vi "WILT Start Stop Button Case.vi"(4 "Semaphore":T1[](array[typedef]), 6 "Dryer Step 4 In":T2 {"Night Cycle Count" format="%04d"; "Day Cycle Count" format="%04d"}, 7 "Agilent Valve and Switch Locations":T4[](array[typedef])=[{"Channel"="301", "Station"="1", "Label"="Water Valve", "Agilent Station"="2", "Data"=0.0}, {"Channel"="302", "Station"="2", "Label"="Water Valve", "Agilent Station"="2", "Data"=0.0}, {"Channel"="303", "Station"="3", "Label"="Water Valve", "Agilent Station"="2", "Data"=0.0}, {"Channel"="304", "Station"="4", "Label"="Water Valve", "Agilent Station"="2", "Data"=0.0}, {"Channel"="305", "Station"="5", "Label"="Water Valve", "Agilent Station"="2", "Data"=0.0}, {"Channel"="306", "Station"="6", "Label"="Water Valve", "Agilent Station"="2", "Data"=0.0}, {"Channel"="307", "Station"="7", "Label"="Water Valve", "Agilent Station"="2", "Data"=0.0}, {"Channel"="308", "Station"="8", "Label"="Water Valve", "Agilent Station"="2", "Data"=0.0}, {"Channel"="309", "Station"="9", "Label"="Water Valve", "Agilent Station"="2", "Data"=0.0}, {"Channel"="310", "Station"="10", "Label"="Water Valve", "Agilent Station"="2", "Data"=0.0}, {"Channel"="311", "Station"="11", "Label"="Water Valve", "Agilent Station"="2", "Data"=0.0}, {"Channel"="312", "Station"="12", "Label"="Water Valve", "Agilent Station"="2", "Data"=0.0}, {"Channel"="313", "Station"="13", "Label"="Water Valve", "Agilent Station"="2", "Data"=0.0}, {"Channel"="314", "Station"="14", "Label"="Water Valve", "Agilent Station"="2", "Data"=0.0}, {"Channel"="315", "Station"="15", "Label"="Water Valve", "Agilent Station"="2", "Data"=0.0}, {"Channel"="316", "Station"="16", "Label"="Water Valve", "Agilent Station"="2", "Data"=0.0}, {"Channel"="317", "Station"="17", "Label"="Water Valve", "Agilent Station"="2", "Data"=0.0}, {"Channel"="318", "Station"="18", "Label"="Water Valve", "Agilent Station"="2", "Data"=0.0}, {"Channel"="319", "Station"="19", "Label"="Water Valve", "Agilent Station"="2", "Data"=0.0}, {"Channel"="320", "Station"="20", "Label"="Water Valve", "Agilent Station"="2", "Data"=0.0}, {"Channel"="101", "Station"="21", "Label"="Water Valve", "Agilent Station"="3", "Data"=0.0}, {"Channel"="102", "Station"="22", "Label"="Water Valve", "Agilent Station"="3", "Data"=0.0}, {"Channel"="103", "Station"="23", "Label"="Water Valve", "Agilent Station"="3", "Data"=0.0}, {"Channel"="104", "Station"="24", "Label"="Water Valve", "Agilent Station"="3", "Data"=0.0}, {"Channel"="105", "Station"="25", "Label"="Water Valve", "Agilent Station"="3", "Data"=0.0}, {"Channel"="106", "Station"="26", "Label"="Water Valve", "Agilent Station"="3", "Data"=0.0}, {"Channel"="107", "Station"="27", "Label"="Water Valve", "Agilent Station"="3", "Data"=0.0}, {"Channel"="108", "Station"="28", "Label"="Water Valve", "Agilent Station"="3", "Data"=0.0}, {"Channel"="109", "Station"="29", "Label"="Water Valve", "Agilent Station"="3", "Data"=0.0}, {"Channel"="110", "Station"="30", "Label"="Water Valve", "Agilent Station"="3", "Data"=0.0}, {"Channel"="111", "Station"="31", "Label"="Water Valve", "Agilent Station"="3", "Data"=0.0}, {"Channel"="112", "Station"="32", "Label"="Water Valve", "Agilent Station"="3", "Data"=0.0}, {"Channel"="101", "Station"="33", "Label"="Water Valve", "Agilent Station"="5", "Data"=0.0}, {"Channel"="102", "Station"="34", "Label"="Water Valve", "Agilent Station"="5", "Data"=0.0}, {"Channel"="103", "Station"="35", "Label"="Water Valve", "Agilent Station"="5", "Data"=0.0}, {"Channel"="104", "Station"="36", "Label"="Water Valve", "Agilent Station"="5", "Data"=0.0}, {"Channel"="105", "Station"="37", "Label"="Water Valve", "Agilent Station"="5", "Data"=0.0}, {"Channel"="106", "Station"="38", "Label"="Water Valve", "Agilent Station"="5", "Data"=0.0}, {"Channel"="107", "Station"="39", "Label"="Water Valve", "Agilent Station"="5", "Data"=0.0}, {"Channel"="108", "Station"="40", "Label"="Water Valve", "Agilent Station"="5", "Data"=0.0}, {"Channel"="109", "Station"="41", "Label"="Water Valve", "Agilent Station"="5", "Data"=0.0}, {"Channel"="110", "Station"="42", "Label"="Water Valve", "Agilent Station"="5", "Data"=0.0}, {"Channel"="111", "Station"="43", "Label"="Water Valve", "Agilent Station"="5", "Data"=0.0}, {"Channel"="112", "Station"="44", "Label"="Water Valve", "Agilent Station"="5", "Data"=0.0}, {"Channel"="113", "Station"="45", "Label"="Water Valve", "Agilent Station"="5", "Data"=0.0}, {"Channel"="114", "Station"="46", "Label"="Water Valve", "Agilent Station"="5", "Data"=0.0}, {"Channel"="115", "Station"="47", "Label"="Water Valve", "Agilent Station"="5", "Data"=0.0}, {"Channel"="116", "Station"="48", "Label"="Water Valve", "Agilent Station"="5", "Data"=0.0}, {"Channel"="117", "Station"="49", "Label"="Water Valve", "Agilent Station"="5", "Data"=0.0}, {"Channel"="118", "Station"="50", "Label"="Water Valve", "Agilent Station"="5", "Data"=0.0}, {"Channel"="119", "Station"="51", "Label"="Water Valve", "Agilent Station"="5", "Data"=0.0}, {"Channel"="120", "Station"="52", "Label"="Water Valve", "Agilent Station"="5", "Data"=0.0}, {"Channel"="201", "Station"="53", "Label"="Water Valve", "Agilent Station"="5", "Data"=0.0}, {"Channel"="202", "Station"="54", "Label"="Water Valve", "Agilent Station"="5", "Data"=0.0}, {"Channel"="203", "Station"="55", "Label"="Water Valve", "Agilent Station"="5", "Data"=0.0}, {"Channel"="204", "Station"="56", "Label"="Water Valve", "Agilent Station"="5", "Data"=0.0}, {"Channel"="301", "Station"="21", "Label"="Start Button", "Agilent Station"="5", "Data"=0.0}, {"Channel"="302", "Station"="22", "Label"="Start Button", "Agilent Station"="5", "Data"=0.0}, {"Channel"="303", "Station"="23", "Label"="Start Button", "Agilent Station"="5", "Data"=0.0}, {"Channel"="304", "Station"="24", "Label"="Start Button", "Agilent Station"="5", "Data"=0.0}, {"Channel"="305", "Station"="25", "Label"="Start Button", "Agilent Station"="5", "Data"=0.0}, {"Channel"="306", "Station"="26", "Label"="Start Button", "Agilent Station"="5", "Data"=0.0}, {"Channel"="307", "Station"="27", "Label"="Start Button", "Agilent Station"="5", "Data"=0.0}, {"Channel"="308", "Station"="28", "Label"="Start Button", "Agilent Station"="5", "Data"=0.0}, {"Channel"="309", "Station"="29", "Label"="Start Button", "Agilent Station"="5", "Data"=0.0}, {"Channel"="310", "Station"="30", "Label"="Start Button", "Agilent Station"="5", "Data"=0.0}, {"Channel"="311", "Station"="31", "Label"="Start Button", "Agilent Station"="5", "Data"=0.0}, {"Channel"="312", "Station"="32", "Label"="Start Button", "Agilent Station"="5", "Data"=0.0}, {"Channel"="101", "Station"="33", "Label"="Start Button", "Agilent Station"="7", "Data"=0.0}, {"Channel"="102", "Station"="34", "Label"="Start Button", "Agilent Station"="7", "Data"=0.0}, {"Channel"="103", "Station"="35", "Label"="Start Button", "Agilent Station"="7", "Data"=0.0}, {"Channel"="104", "Station"="36", "Label"="Start Button", "Agilent Station"="7", "Data"=0.0}, {"Channel"="105", "Station"="37", "Label"="Start Button", "Agilent Station"="7", "Data"=0.0}, {"Channel"="106", "Station"="38", "Label"="Start Button", "Agilent Station"="7", "Data"=0.0}, {"Channel"="107", "Station"="39", "Label"="Start Button", "Agilent Station"="7", "Data"=0.0}, {"Channel"="108", "Station"="40", "Label"="Start Button", "Agilent Station"="7", "Data"=0.0}, {"Channel"="109", "Station"="41", "Label"="Start Button", "Agilent Station"="7", "Data"=0.0}, {"Channel"="110", "Station"="42", "Label"="Start Button", "Agilent Station"="7", "Data"=0.0}, {"Channel"="111", "Station"="43", "Label"="Start Button", "Agilent Station"="7", "Data"=0.0}, {"Channel"="112", "Station"="44", "Label"="Start Button", "Agilent Station"="7", "Data"=0.0}], 8 "Error In":errorcluster, 9 "Final Start Presses":i32=2, 10 "Station Number":u32, 11 "Step 3 Input in":T6) -> (0 "Error Out":errorcluster, 3 "Step 3 Input out":T6)   [LabVIEW 2016]
uses:
  Type Definitions/WILT Station Test State Cluster.ctl
  Type Definitions/WILT Dryer Test State.ctl
  Type Definitions/WILT Agilent Channel Definition.ctl
  Type Definitions/WILT Dryer.ctl
  Type Definitions/WILT Dryer Details.ctl
  Type Definitions/WILT DAQ Data.ctl
  Type Definitions/WILT Water Valve Test Type.ctl
  Type Definitions/WILT Switch Search.ctl
panel:
  # "Day"
  # "Night"
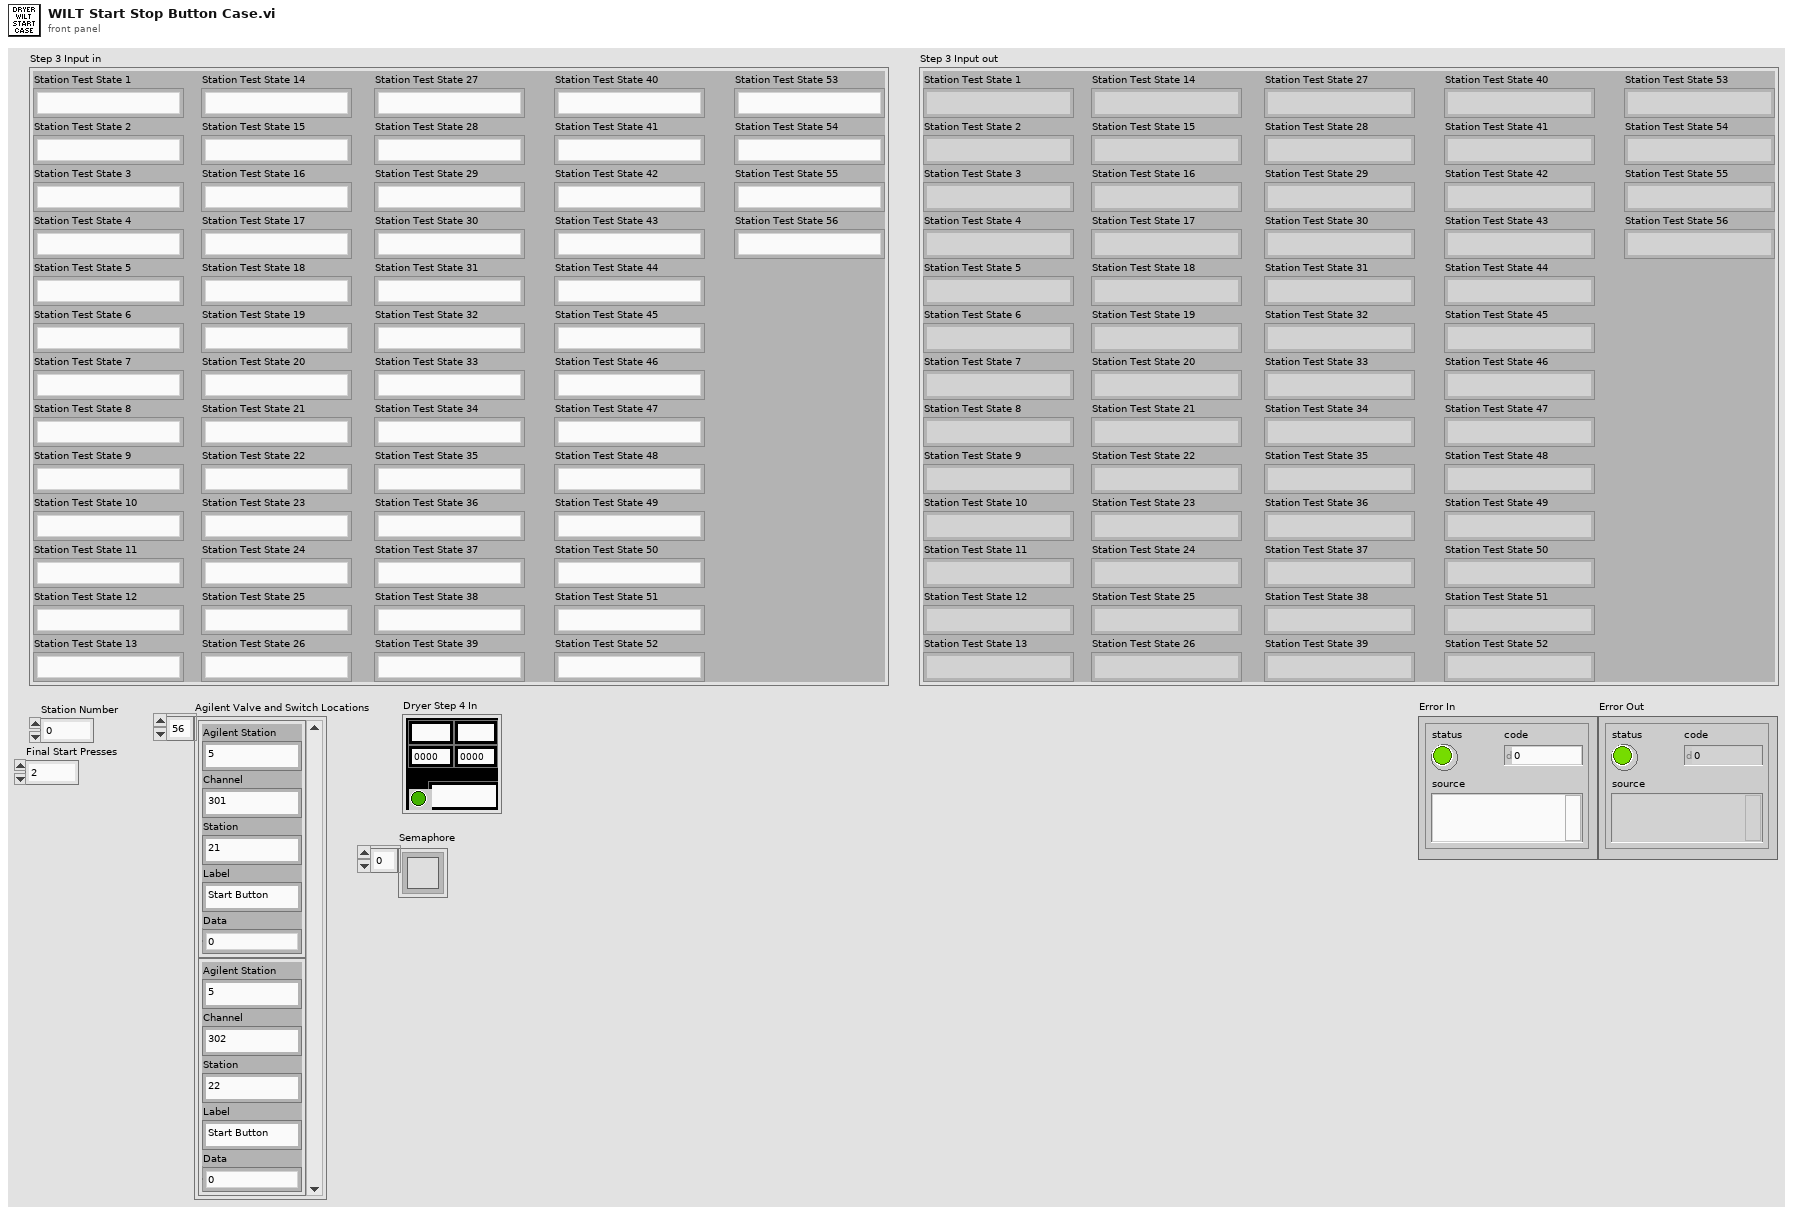
[diagram p1: front panel]
types:
  T1 = typedef "Semaphore RefNum" = refnum<k1>
  T2 = typedef "WILT Dryer.ctl" = cluster{"Lab ID":string, "Day Cycle Count":i32, "Station Label":string, "Dryer Details":T3, "Status Color":u32, "Invisible Button":bool, "Night Cycle Count":i32, "Station Index":i32, "Cycle Index":string, "Audit Alert":bool, "Agilent Channel Definition":T4, "DAQ Data":T5}
  T3 = typedef "WILT Dryer Details.ctl" = cluster{"Station":string, "Lab ID":string, "TR Number":string}
  T4 = typedef "WILT Agilent Channel Definition.ctl" = cluster{"Channel":string, "Station":string, "Label":string, "Agilent Station":string, "Data":dbl}
  T5 = typedef "WILT DAQ Data.ctl" = cluster{"L1 Current":dbl, "L2 Current":dbl, "Temperature  Deg F (TC)":dbl, "Volts":dbl, "Volts (208)":dbl, "SW (208)":dbl}
  T6 = typedef "WILT Station Test State Cluster.ctl" = cluster{"Station Test State 1":T7, "Station Test State 2":T7, "Station Test State 3":T7, "Station Test State 4":T7, "Station Test State 5":T7, "Station Test State 6":T7, "Station Test State 7":T7, "Station Test State 8":T7, "Station Test State 9":T7, "Station Test State 10":T7, "Station Test State 11":T7, "Station Test State 12":T7, "Station Test State 13":T7, "Station Test State 14":T7, "Station Test State 15":T7, "Station Test State 16":T7, "Station Test State 17":T7, "Station Test State 18":T7, "Station Test State 19":T7, "Station Test State 20":T7, "Station Test State 21":T7, "Station Test State 22":T7, "Station Test State 23":T7, "Station Test State 24":T7, "Station Test State 25":T7, "Station Test State 26":T7, "Station Test State 27":T7, "Station Test State 28":T7, "Station Test State 29":T7, "Station Test State 30":T7, "Station Test State 31":T7, "Station Test State 32":T7, "Station Test State 33":T7, "Station Test State 34":T7, "Station Test State 35":T7, "Station Test State 36":T7, "Station Test State 37":T7, "Station Test State 38":T7, "Station Test State 39":T7, "Station Test State 40":T7, "Station Test State 41":T7, "Station Test State 42":T7, "Station Test State 43":T7, "Station Test State 44":T7, "Station Test State 45":T7, "Station Test State 46":T7, "Station Test State 47":T7, "Station Test State 48":T7, "Station Test State 49":T7, "Station Test State 50":T7, "Station Test State 51":T7, "Station Test State 52":T7, "Station Test State 53":T7, "Station Test State 54":T7, "Station Test State 55":T7, "Station Test State 56":T7}
  T7 = typedef "WILT Dryer Test State.ctl" = enum16{"No Serial Number", "Waiting for Dryer To Start", "Drying Clothes", "Water Injection 1 (On)", "Water Injection 1 Timer", "Water Injection 1 (Off)", "Pause Dryer", "Sending Start Stop CMD", "Pause Dryer 2", "Sending Start Stop CMD 2", "Drying Clothes 2", "Water Injection 2 (On)", "Water Injection 2 Timer", "Water Injection 2 (Off)", "Drying Clothes 3", "Cooling Down", "Sending Start Stop CMD 3", "Increment Cycle"}
  T8 = typedef "WILT Switch Search.ctl" = string
  T9 = typedef "WILT Water Valve Test Type.ctl" = enum16{"Cycle Valve Control", "Full Valve Control"}
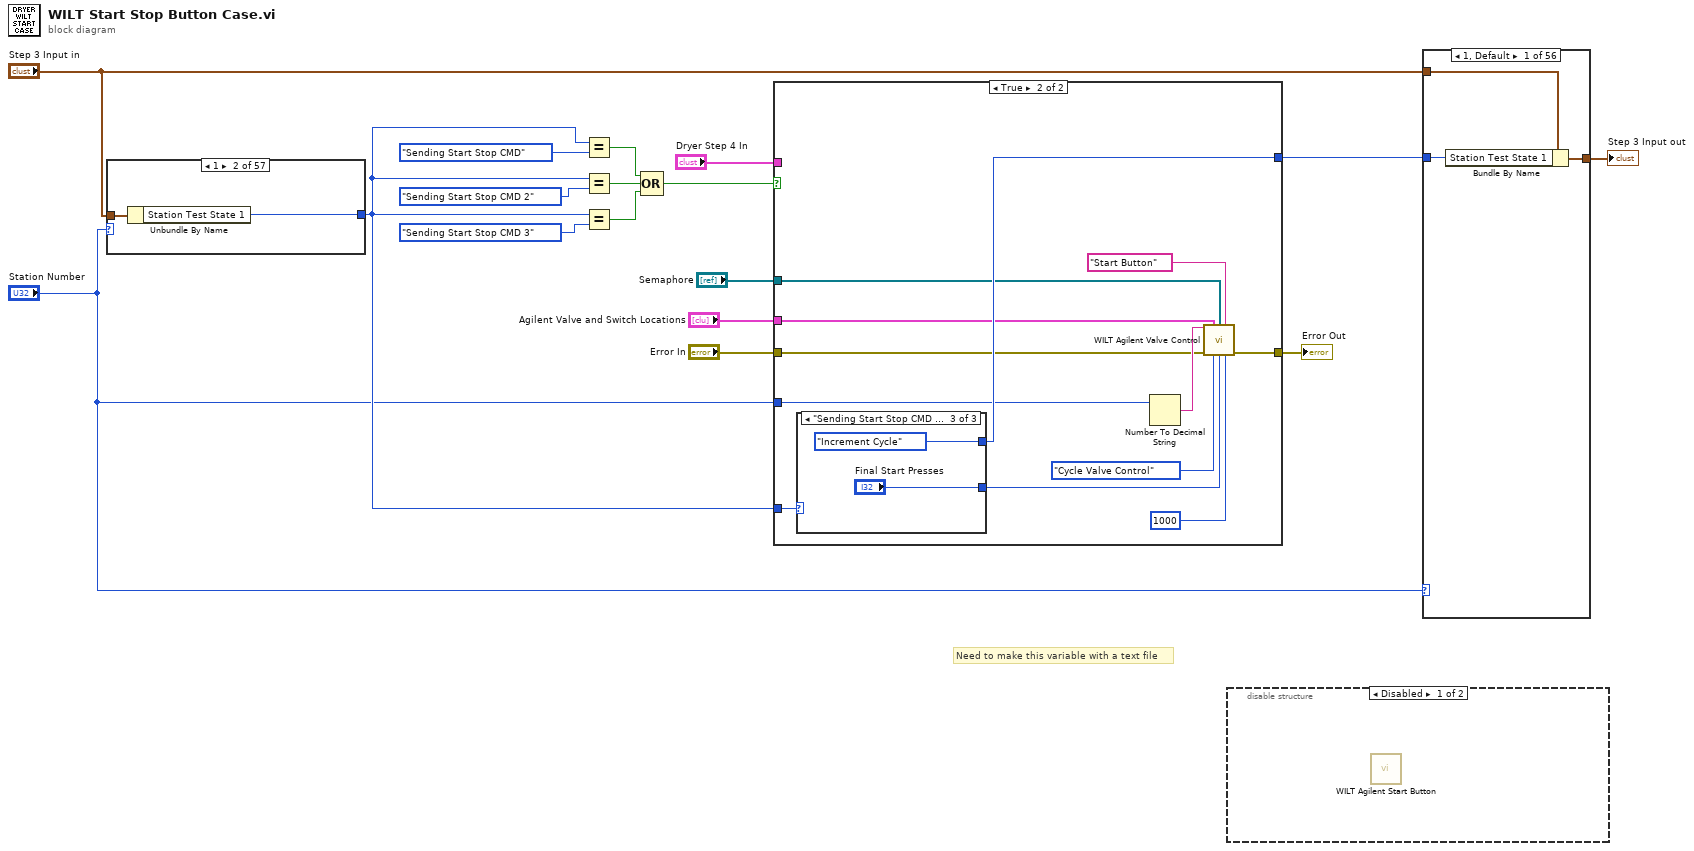
[diagram p0: block diagram]
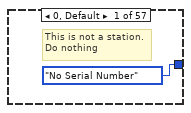
[diagram p3: hidden frame]
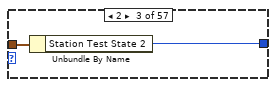
[diagram p4: hidden frame]
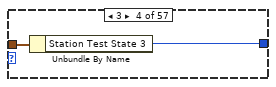
[diagram p5: hidden frame]
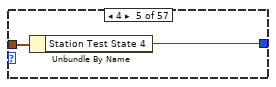
[diagram p6: hidden frame]
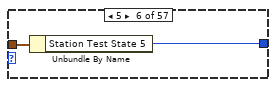
[diagram p7: hidden frame]
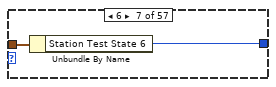
[diagram p8: hidden frame]
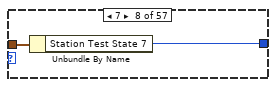
[diagram p9: hidden frame]
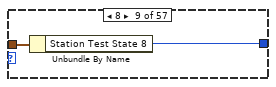
[diagram p10: hidden frame]
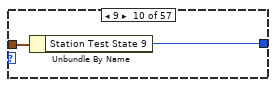
[diagram p11: hidden frame]
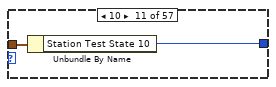
[diagram p12: hidden frame]
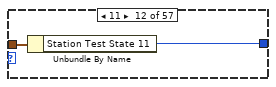
[diagram p13: hidden frame]
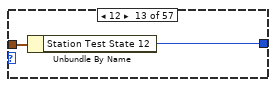
[diagram p14: hidden frame]
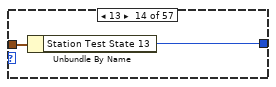
[diagram p15: hidden frame]
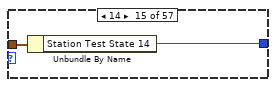
[diagram p16: hidden frame]
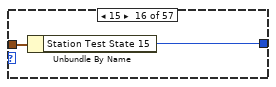
[diagram p17: hidden frame]
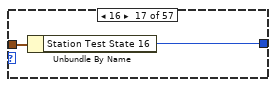
[diagram p18: hidden frame]
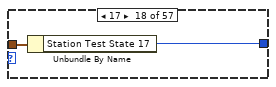
[diagram p19: hidden frame]
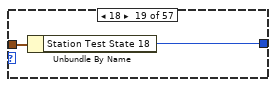
[diagram p20: hidden frame]
diagram:
  # "Need to make this variable with a text file"
  n1 = case shown="1" "Station Number" {
    tunnel: "Step 3 Input in" -> [_ w20 w22 w24 w26 w28 w30 w32 w34 w36 w38 w40 w42 w44 w46 w48 w50 w52 w54 w56 w58 w60 w62 w64 w66 w68 w70 w72 w74 w76 w78 w80 w82 w84 w86 w88 w90 w92 w94 w96 w98 w100 w102 w104 w106 w108 w110 w112 w114 w116 w118 w120 w122 w124 w126 w128 w130]
    tunnel: [WILT_Dryer_Test_State."No Serial Number" ("Station Test State 56") w19 w21 w23 w25 w27 w29 w31 w33 w35 w37 w39 w41 w43 w45 w47 w49 w51 w53 w55 w57 w59 w61 w63 w65 w67 w69 w71 w73 w75 w77 w79 w81 w83 w85 w87 w89 w91 w93 w95 w97 w99 w101 w103 w105 w107 w109 w111 w113 w115 w117 w119 w121 w123 w125 w127 w129] -> w6
    frame 0, Default {
      # "This is not a station.\nDo nothing"
    }
    frame 1 {
      n2 = Unbundle By Name(w20) -> ("Station Test State 1"=w19:T7)
    }
    frame 2 {
      n3 = Unbundle By Name(w22) -> ("Station Test State 2"=w21:T7)
    }
    frame 3 {
      n4 = Unbundle By Name(w24) -> ("Station Test State 3"=w23:T7)
    }
    frame 4 {
      n5 = Unbundle By Name(w26) -> ("Station Test State 4"=w25:T7)
    }
    frame 5 {
      n6 = Unbundle By Name(w28) -> ("Station Test State 5"=w27:T7)
    }
    frame 6 {
      n7 = Unbundle By Name(w30) -> ("Station Test State 6"=w29:T7)
    }
    frame 7 {
      n8 = Unbundle By Name(w32) -> ("Station Test State 7"=w31:T7)
    }
    frame 8 {
      n9 = Unbundle By Name(w34) -> ("Station Test State 8"=w33:T7)
    }
    frame 9 {
      n10 = Unbundle By Name(w36) -> ("Station Test State 9"=w35:T7)
    }
    frame 10 {
      n11 = Unbundle By Name(w38) -> ("Station Test State 10"=w37:T7)
    }
    frame 11 {
      n12 = Unbundle By Name(w40) -> ("Station Test State 11"=w39:T7)
    }
    frame 12 {
      n13 = Unbundle By Name(w42) -> ("Station Test State 12"=w41:T7)
    }
    frame 13 {
      n14 = Unbundle By Name(w44) -> ("Station Test State 13"=w43:T7)
    }
    frame 14 {
      n15 = Unbundle By Name(w46) -> ("Station Test State 14"=w45:T7)
    }
    frame 15 {
      n16 = Unbundle By Name(w48) -> ("Station Test State 15"=w47:T7)
    }
    frame 16 {
      n17 = Unbundle By Name(w50) -> ("Station Test State 16"=w49:T7)
    }
    frame 17 {
      n18 = Unbundle By Name(w52) -> ("Station Test State 17"=w51:T7)
    }
    frame 18 {
      n19 = Unbundle By Name(w54) -> ("Station Test State 18"=w53:T7)
    }
    frame 19 {
      n20 = Unbundle By Name(w56) -> ("Station Test State 19"=w55:T7)
    }
    frame 20 {
      n21 = Unbundle By Name(w58) -> ("Station Test State 20"=w57:T7)
    }
    frame 21 {
      n22 = Unbundle By Name(w60) -> ("Station Test State 21"=w59:T7)
    }
    frame 22 {
      n23 = Unbundle By Name(w62) -> ("Station Test State 22"=w61:T7)
    }
    frame 23 {
      n24 = Unbundle By Name(w64) -> ("Station Test State 23"=w63:T7)
    }
    frame 24 {
      n25 = Unbundle By Name(w66) -> ("Station Test State 24"=w65:T7)
    }
    frame 25 {
      n26 = Unbundle By Name(w68) -> ("Station Test State 25"=w67:T7)
    }
    frame 26 {
      n27 = Unbundle By Name(w70) -> ("Station Test State 26"=w69:T7)
    }
    frame 27 {
      n28 = Unbundle By Name(w72) -> ("Station Test State 27"=w71:T7)
    }
    frame 28 {
      n29 = Unbundle By Name(w74) -> ("Station Test State 28"=w73:T7)
    }
    frame 29 {
      n30 = Unbundle By Name(w76) -> ("Station Test State 29"=w75:T7)
    }
    frame 30 {
      n31 = Unbundle By Name(w78) -> ("Station Test State 30"=w77:T7)
    }
    frame 31 {
      n32 = Unbundle By Name(w80) -> ("Station Test State 31"=w79:T7)
    }
    frame 32 {
      n33 = Unbundle By Name(w82) -> ("Station Test State 32"=w81:T7)
    }
    frame 33 {
      n34 = Unbundle By Name(w84) -> ("Station Test State 33"=w83:T7)
    }
    frame 34 {
      n35 = Unbundle By Name(w86) -> ("Station Test State 34"=w85:T7)
    }
    frame 35 {
      n36 = Unbundle By Name(w88) -> ("Station Test State 35"=w87:T7)
    }
    frame 36 {
      n37 = Unbundle By Name(w90) -> ("Station Test State 36"=w89:T7)
    }
    frame 37 {
      n38 = Unbundle By Name(w92) -> ("Station Test State 37"=w91:T7)
    }
    frame 38 {
      n39 = Unbundle By Name(w94) -> ("Station Test State 38"=w93:T7)
    }
    frame 39 {
      n40 = Unbundle By Name(w96) -> ("Station Test State 39"=w95:T7)
    }
    frame 40 {
      n41 = Unbundle By Name(w98) -> ("Station Test State 40"=w97:T7)
    }
    frame 41 {
      n42 = Unbundle By Name(w100) -> ("Station Test State 41"=w99:T7)
    }
    frame 42 {
      n43 = Unbundle By Name(w102) -> ("Station Test State 42"=w101:T7)
    }
    frame 43 {
      n44 = Unbundle By Name(w104) -> ("Station Test State 43"=w103:T7)
    }
    frame 44 {
      n45 = Unbundle By Name(w106) -> ("Station Test State 44"=w105:T7)
    }
    frame 45 {
      n46 = Unbundle By Name(w108) -> ("Station Test State 45"=w107:T7)
    }
    frame 46 {
      n47 = Unbundle By Name(w110) -> ("Station Test State 46"=w109:T7)
    }
    frame 47 {
      n48 = Unbundle By Name(w112) -> ("Station Test State 47"=w111:T7)
    }
    frame 48 {
      n49 = Unbundle By Name(w114) -> ("Station Test State 48"=w113:T7)
    }
    frame 49 {
      n50 = Unbundle By Name(w116) -> ("Station Test State 49"=w115:T7)
    }
    frame 50 {
      n51 = Unbundle By Name(w118) -> ("Station Test State 50"=w117:T7)
    }
    frame 51 {
      n52 = Unbundle By Name(w120) -> ("Station Test State 51"=w119:T7)
    }
    frame 52 {
      n53 = Unbundle By Name(w122) -> ("Station Test State 52"=w121:T7)
    }
    frame 53 {
      n54 = Unbundle By Name(w124) -> ("Station Test State 53"=w123:T7)
    }
    frame 54 {
      n55 = Unbundle By Name(w126) -> ("Station Test State 54"=w125:T7)
    }
    frame 55 {
      n56 = Unbundle By Name(w128) -> ("Station Test State 55"=w127:T7)
    }
    frame 56 {
      n57 = Unbundle By Name(w130) -> ("Station Test State 56"=w129:T7)
    }
  }
  n58 = Equal?(x=w6, y=WILT_Dryer_Test_State."Sending Start Stop CMD") -> (x = y?=w14:bool)
  n59 = Equal?(x=w6, y=WILT_Dryer_Test_State."Sending Start Stop CMD 2") -> (x = y?=w15:bool)
  n60 = Equal?(x=w6, y=WILT_Dryer_Test_State."Sending Start Stop CMD 3") -> (x = y?=w16:bool)
  n61 = Compound Arithmetic op=OR(w14, w15, w16) -> (w17:bool)
  n62 = case shown="True" w17 {
    tunnel: "Station Number" -> [_ w138]
    tunnel: [WILT_Dryer_Test_State."Waiting for Dryer To Start" ("Station Test State 56") w143] -> w8
    tunnel: w6 -> [_ w144]
    tunnel: "Error In" -> [w131 w139]
    tunnel: [w131 w137] -> w9
    tunnel: "Agilent Valve and Switch Locations" -> [_ w133]
    tunnel: "Dryer Step 4 In" -> [_ _]
    tunnel: "Semaphore" -> [_ w134]
    frame False {
    }
    frame True {
      n63 = case shown="\"Sending Start Stop CMD 3\"" w144 {
        tunnel: [1 ("Number Of Cycles") 1 ("Number Of Cycles") "Final Start Presses"] -> w136
        tunnel: [WILT_Dryer_Test_State."Pause Dryer 2" ("Station Test State 56") WILT_Dryer_Test_State."Drying Clothes 2" ("Station Test State 56") WILT_Dryer_Test_State."Increment Cycle" ("Station Test State 56")] -> w143
        frame "Sending Start Stop CMD", Default {
        }
        frame "Sending Start Stop CMD 2" {
        }
        frame "Sending Start Stop CMD 3" {
        }
      }
      n64 = Number To Decimal String(number=w138) -> (decimal integer string=w142:string)  [unwired: 1 in]
      n65 = call "WILT Agilent Valve Control.vi"("Station In"=w142, "Agilent Channels In"=w133, "Semaphore"=w134, "Search"=T8 "Start Button", "error in (no error)"=w139, "Test Type"=WILT_Water_Valve_Test_Type."Cycle Valve Control", "Number Of Cycles"=w136, "Cycle Time (mS)"=u32 1000) -> ("error out"=w137:errorcluster)  [unwired: 5 in, 2 out]
    }
  }
  "Error Out" <- w9
  n66 = disable-structure shown="Disabled" {
    frame Disabled {
      n67 = call "WILT Agilent Start Button.vi"() -> ()  [unwired: 15 in, 1 out]
    }
    frame Enabled {
    }
  }
  n68 = case shown="1, Default" "Station Number" {
    tunnel: "Step 3 Input in" -> [w153 w156 w159 w162 w165 w168 w171 w174 w177 w180 w183 w186 w189 w192 w195 w198 w201 w204 w207 w210 w213 w216 w219 w222 w225 w228 w231 w234 w237 w240 w243 w246 w249 w252 w255 w258 w261 w264 w267 w270 w273 w276 w279 w282 w285 w288 w291 w294 w297 w300 w303 w306 w309 w312 w315 w318]
    tunnel: w8 -> [w152 w154 w157 w160 w163 w166 w169 w172 w175 w178 w181 w184 w187 w190 w193 w196 w199 w202 w205 w208 w211 w214 w217 w220 w223 w226 w229 w232 w235 w238 w241 w244 w247 w250 w253 w256 w259 w262 w265 w268 w271 w274 w277 w280 w283 w286 w289 w292 w295 w298 w301 w304 w307 w310 w313 w316]
    tunnel: [w151 w155 w158 w161 w164 w167 w170 w173 w176 w179 w182 w185 w188 w191 w194 w197 w200 w203 w206 w209 w212 w215 w218 w221 w224 w227 w230 w233 w236 w239 w242 w245 w248 w251 w254 w257 w260 w263 w266 w269 w272 w275 w278 w281 w284 w287 w290 w293 w296 w299 w302 w305 w308 w311 w314 w317] -> w7
    frame 1, Default {
      n69 = Bundle By Name(cluster=w153, "Station Test State 1"=w152) -> (w151:T6)
    }
    frame 2 {
      n70 = Bundle By Name(cluster=w156, "Station Test State 2"=w154) -> (w155:T6)
    }
    frame 3 {
      n71 = Bundle By Name(cluster=w159, "Station Test State 3"=w157) -> (w158:T6)
    }
    frame 4 {
      n72 = Bundle By Name(cluster=w162, "Station Test State 4"=w160) -> (w161:T6)
    }
    frame 5 {
      n73 = Bundle By Name(cluster=w165, "Station Test State 5"=w163) -> (w164:T6)
    }
    frame 6 {
      n74 = Bundle By Name(cluster=w168, "Station Test State 6"=w166) -> (w167:T6)
    }
    frame 7 {
      n75 = Bundle By Name(cluster=w171, "Station Test State 7"=w169) -> (w170:T6)
    }
    frame 8 {
      n76 = Bundle By Name(cluster=w174, "Station Test State 8"=w172) -> (w173:T6)
    }
    frame 9 {
      n77 = Bundle By Name(cluster=w177, "Station Test State 9"=w175) -> (w176:T6)
    }
    frame 10 {
      n78 = Bundle By Name(cluster=w180, "Station Test State 10"=w178) -> (w179:T6)
    }
    frame 11 {
      n79 = Bundle By Name(cluster=w183, "Station Test State 11"=w181) -> (w182:T6)
    }
    frame 12 {
      n80 = Bundle By Name(cluster=w186, "Station Test State 12"=w184) -> (w185:T6)
    }
    frame 13 {
      n81 = Bundle By Name(cluster=w189, "Station Test State 13"=w187) -> (w188:T6)
    }
    frame 14 {
      n82 = Bundle By Name(cluster=w192, "Station Test State 14"=w190) -> (w191:T6)
    }
    frame 15 {
      n83 = Bundle By Name(cluster=w195, "Station Test State 15"=w193) -> (w194:T6)
    }
    frame 16 {
      n84 = Bundle By Name(cluster=w198, "Station Test State 16"=w196) -> (w197:T6)
    }
    frame 17 {
      n85 = Bundle By Name(cluster=w201, "Station Test State 17"=w199) -> (w200:T6)
    }
    frame 18 {
      n86 = Bundle By Name(cluster=w204, "Station Test State 18"=w202) -> (w203:T6)
    }
    frame 19 {
      n87 = Bundle By Name(cluster=w207, "Station Test State 19"=w205) -> (w206:T6)
    }
    frame 20 {
      n88 = Bundle By Name(cluster=w210, "Station Test State 20"=w208) -> (w209:T6)
    }
    frame 21 {
      n89 = Bundle By Name(cluster=w213, "Station Test State 21"=w211) -> (w212:T6)
    }
    frame 22 {
      n90 = Bundle By Name(cluster=w216, "Station Test State 22"=w214) -> (w215:T6)
    }
    frame 23 {
      n91 = Bundle By Name(cluster=w219, "Station Test State 23"=w217) -> (w218:T6)
    }
    frame 24 {
      n92 = Bundle By Name(cluster=w222, "Station Test State 24"=w220) -> (w221:T6)
    }
    frame 25 {
      n93 = Bundle By Name(cluster=w225, "Station Test State 25"=w223) -> (w224:T6)
    }
    frame 26 {
      n94 = Bundle By Name(cluster=w228, "Station Test State 26"=w226) -> (w227:T6)
    }
    frame 27 {
      n95 = Bundle By Name(cluster=w231, "Station Test State 27"=w229) -> (w230:T6)
    }
    frame 28 {
      n96 = Bundle By Name(cluster=w234, "Station Test State 28"=w232) -> (w233:T6)
    }
    frame 29 {
      n97 = Bundle By Name(cluster=w237, "Station Test State 29"=w235) -> (w236:T6)
    }
    frame 30 {
      n98 = Bundle By Name(cluster=w240, "Station Test State 30"=w238) -> (w239:T6)
    }
    frame 31 {
      n99 = Bundle By Name(cluster=w243, "Station Test State 31"=w241) -> (w242:T6)
    }
    frame 32 {
      n100 = Bundle By Name(cluster=w246, "Station Test State 32"=w244) -> (w245:T6)
    }
    frame 33 {
      n101 = Bundle By Name(cluster=w249, "Station Test State 33"=w247) -> (w248:T6)
    }
    frame 34 {
      n102 = Bundle By Name(cluster=w252, "Station Test State 34"=w250) -> (w251:T6)
    }
    frame 35 {
      n103 = Bundle By Name(cluster=w255, "Station Test State 35"=w253) -> (w254:T6)
    }
    frame 36 {
      n104 = Bundle By Name(cluster=w258, "Station Test State 36"=w256) -> (w257:T6)
    }
    frame 37 {
      n105 = Bundle By Name(cluster=w261, "Station Test State 37"=w259) -> (w260:T6)
    }
    frame 38 {
      n106 = Bundle By Name(cluster=w264, "Station Test State 38"=w262) -> (w263:T6)
    }
    frame 39 {
      n107 = Bundle By Name(cluster=w267, "Station Test State 39"=w265) -> (w266:T6)
    }
    frame 40 {
      n108 = Bundle By Name(cluster=w270, "Station Test State 40"=w268) -> (w269:T6)
    }
    frame 41 {
      n109 = Bundle By Name(cluster=w273, "Station Test State 41"=w271) -> (w272:T6)
    }
    frame 42 {
      n110 = Bundle By Name(cluster=w276, "Station Test State 42"=w274) -> (w275:T6)
    }
    frame 43 {
      n111 = Bundle By Name(cluster=w279, "Station Test State 43"=w277) -> (w278:T6)
    }
    frame 44 {
      n112 = Bundle By Name(cluster=w282, "Station Test State 44"=w280) -> (w281:T6)
    }
    frame 45 {
      n113 = Bundle By Name(cluster=w285, "Station Test State 45"=w283) -> (w284:T6)
    }
    frame 46 {
      n114 = Bundle By Name(cluster=w288, "Station Test State 46"=w286) -> (w287:T6)
    }
    frame 47 {
      n115 = Bundle By Name(cluster=w291, "Station Test State 47"=w289) -> (w290:T6)
    }
    frame 48 {
      n116 = Bundle By Name(cluster=w294, "Station Test State 48"=w292) -> (w293:T6)
    }
    frame 49 {
      n117 = Bundle By Name(cluster=w297, "Station Test State 49"=w295) -> (w296:T6)
    }
    frame 50 {
      n118 = Bundle By Name(cluster=w300, "Station Test State 50"=w298) -> (w299:T6)
    }
    frame 51 {
      n119 = Bundle By Name(cluster=w303, "Station Test State 51"=w301) -> (w302:T6)
    }
    frame 52 {
      n120 = Bundle By Name(cluster=w306, "Station Test State 52"=w304) -> (w305:T6)
    }
    frame 53 {
      n121 = Bundle By Name(cluster=w309, "Station Test State 53"=w307) -> (w308:T6)
    }
    frame 54 {
      n122 = Bundle By Name(cluster=w312, "Station Test State 54"=w310) -> (w311:T6)
    }
    frame 55 {
      n123 = Bundle By Name(cluster=w315, "Station Test State 55"=w313) -> (w314:T6)
    }
    frame 56 {
      n124 = Bundle By Name(cluster=w318, "Station Test State 56"=w316) -> (w317:T6)
    }
  }
  "Step 3 Input out" <- w7
